vi "load_class.vi"(7 "config in":T1, 8 "error in (no error)":errorcluster) -> (0 "error out":errorcluster, 2 "forced_default":bool, 3 "lv-builder":refnum<class "lv-builder.lvclass">)   [LabVIEW 2015, in "lv-build-interface.lvlib"]
uses:
  lv-build-interface.lvlib
  lv-builder/lv-builder.lvclass
  lv-build/public/_controls/configuration.ctl
  lv-builder-default/lv-builder-default.lvclass
  lv-builder/lv-builder.lvlib
  lv-build/lv-build.lvlib
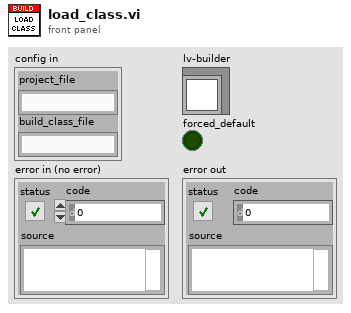
[diagram p1: front panel]
types:
  T1 = typedef "lv-build.lvlib/configuration.ctl" = cluster{"project_file":string, "build_class_file":string}
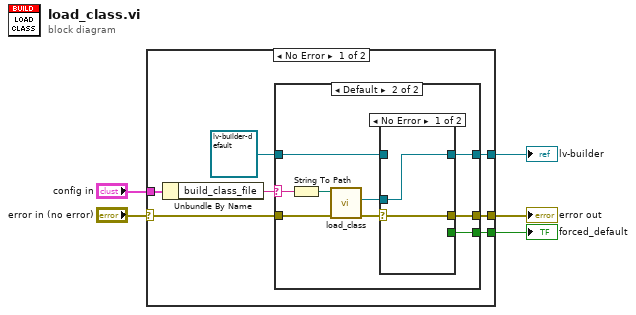
[diagram p0: block diagram]
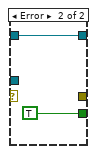
[diagram p3: hidden frame]
diagram:
  n1 = case shown="No Error" "error in (no error)" {
    selector: "error in (no error)" -> [w11 w28]
    tunnel: "config in" -> [w12 _]
    tunnel: [w10 w28] -> w4
    tunnel: [w9 _] -> w3
    tunnel: [w6 _] -> w1
    frame No Error {
      n2 = Unbundle By Name(w12) -> ("build_class_file"=w8:string)
      n3 = case shown="Default" w8 {
        selector: w8 -> [_ w23]
        tunnel: w11 -> [w14 w21]
        tunnel: [w14 w18] -> w10
        tunnel: [w13 w17] -> w9
        tunnel: refnum<class "lv-builder-default.lvclass"> refnum ("lv-builder-default.lvlib:lv-builder-default.lvclass") -> [w13 w16]
        tunnel: [_ w15] -> w6
        frame "" {
        }
        frame Default {
          n4 = String To Path(string=w23) -> (path=w22:path)
          n5 = call "load_class.vi"("error in (no error)"=w21, "builder_class in"=w22) -> ("error out"=w19:errorcluster, "lv_builder"=w20:refnum<class "lv-builder.lvclass">)  [unwired: 6 in, 2 out]
          n6 = case shown="No Error" w19 {
            selector: w19 -> [w25 _]
            tunnel: w20 -> [w24 _]
            tunnel: [w25 _] -> w18
            tunnel: [w24 w27] -> w17
            tunnel: w16 -> [_ w27]
            tunnel: [_ TRUE] -> w15
            frame No Error {
            }
            frame Error {
            }
          }
        }
      }
    }
    frame Error {
    }
  }
  "lv-builder" <- w3
  "error out" <- w4
  "forced_default" <- w1
